vi "write coils.vi"(6 "Ignore Mask?":bool, 7 "Write Mask":bool[](array[boolean]), 8 "error in (no error)":errorcluster, 9 "Channel Data":T1[](array[typedef]), 10 "Values":dbl[](array[numeric]), 11 "Modbus API.lvlibp:Modbus API":refnum<class "Modbus API.lvclass">) -> (0 "error out":errorcluster)   [LabVIEW 2015, in "Modbus Master Engine.lvlib"]
uses:
  Modbus Master Engine.lvlib
  Shared/Controls/Data Model/Channel.ctl
  System Explorer/SubVIs/Modbus Type.ctl
  <vilib>/NI Veristand/Custom Device API/Custom Device Channel Type.ctl
  Shared/Controls/Data Model/Mapping.ctl
  Shared/Controls/Data Model/DataType.ctl
  <vilib>/NI Veristand/Custom Device API/Custom Device Item Ref.ctl
  Modbus API.lvlibp/API/Modbus API.lvclass
  Shared/Modbus Master Shared.lvlib
  <vilib>/NI VeriStand/Custom Device API/Custom Device API.lvlib
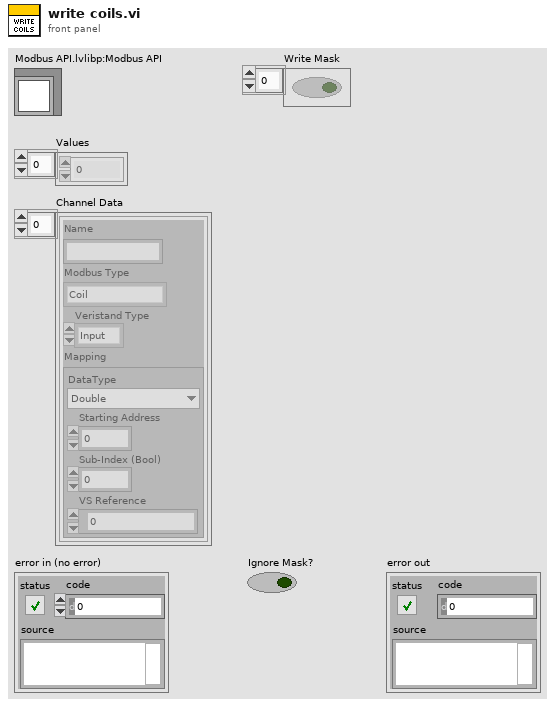
[diagram p1: front panel]
types:
  T1 = typedef "Modbus Master Shared.lvlib/Channel.ctl" = cluster{"Name":string, "Modbus Type":T2, "Veristand Type":T3, "Mapping":T4}
  T2 = typedef "Modbus Master Shared.lvlib/Modbus Type.ctl" = enum16{"Coil", "Discrete Input", "Holding Register", "Input Register"}
  T3 = typedef "Custom Device API.lvlib/Custom Device Channel Type.ctl" = enum16{"Input", "Output"}
  T4 = typedef "Modbus Master Shared.lvlib/Mapping.ctl" = cluster{"DataType":T5, "Starting Address":u16, "Sub-Index (Bool)":u16, "VS Reference":T6}
  T5 = typedef "Modbus Master Shared.lvlib/DataType.ctl" = enum16{"Double", "Single", "I64", "I32", "I16", "I8", "U64", "U32", "U16", "U8", "Boolean"}
  T6 = typedef "Custom Device API.lvlib/Custom Device Item Ref.ctl" = u64
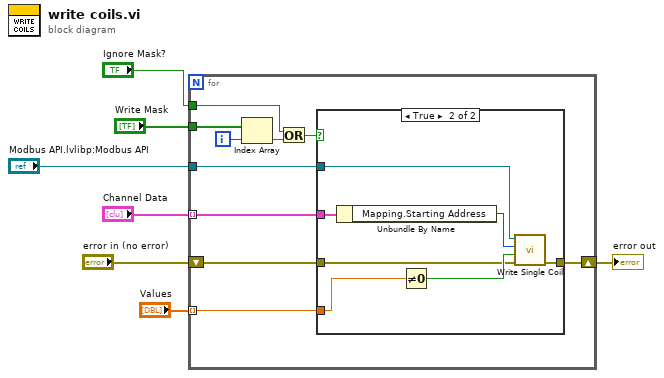
[diagram p0: block diagram]
diagram:
  n1 = for {
    tunnel: "Modbus API.lvlibp:Modbus API" -> [w17]
    tunnel: "Values" -> [w15] mode=indexing
    shift-right: [w13] -> w5
    shift-left: "error in (no error)" -> [w16]
    tunnel: "Write Mask" -> [w10]
    tunnel: "Channel Data" -> [w14] mode=indexing
    tunnel: "Ignore Mask?" -> [w12]
    i -> [w9]
    n2 = Index Array(array=w10, index=w9) -> (element=w8:bool)
    n3 = Or(x=w12, y=w8) -> (x .or. y?=w11:bool)
    n4 = case shown="True" w11 {
      tunnel: w17 -> [_ w20]
      tunnel: w16 -> [w18 w21]
      tunnel: [w18 w19] -> w13
      tunnel: w15 -> [_ w25]
      tunnel: w14 -> [_ w24]
      frame False {
      }
      frame True {
        n5 = Unbundle By Name(w24) -> ("Mapping.Starting Address"=w23:u16)
        n6 = Not Equal To 0?(x=w25) -> (x != 0?=w22:bool)
        n7 = call-dynamic "Write Single Coil.vi"("error in"=w21, "coil to write"=w22, "address"=w23, "Modbus instance in"=w20) -> ("error out"=w19:errorcluster)  [unwired: 6 in, 1 out]
      }
    }
  }
  "error out" <- w5
